vi "RESTful Configure Service Settings.vi"(4 "Number VIs":i32, 6 "Number of Routing Templates":i32, 7 "target reference":refnum<vi>, 8 "error in":errorcluster, 9 "RESTful VI service information":T3, 10 "AMQP Ini In":string="#Service Information", 11 "Master Text In":string="#Service Information") -> (0 "error out":errorcluster, 1 "Service attributes":T1[](array[typedef]), 2 "AMQP Ini Out":string="#Service Information", 3 "Master Text Out":string="#Service Information", 5 "dup target reference":refnum<vi>)   [LabVIEW 2020]
doc: "This VI configure the global settings for the webservices INI file."
uses:
  <vilib>/AppBuilder/Engine/RESTful INI Generator/AB_RESTful_ServiceInfo.ctl
  <vilib>/AppBuilder/AB_Classes/RESTful/AB_RESTful_ServiceAttribute.ctl
  <vilib>/AppBuilder/AB_Classes/RESTful/AB_RESTful_ServiceAttributeType.ctl
  <vilib>/AppBuilder/Engine/RESTful INI Generator/AB_RESTful_ServiceType.ctl
  <vilib>/Utility/error.llb/whitespace.ctl
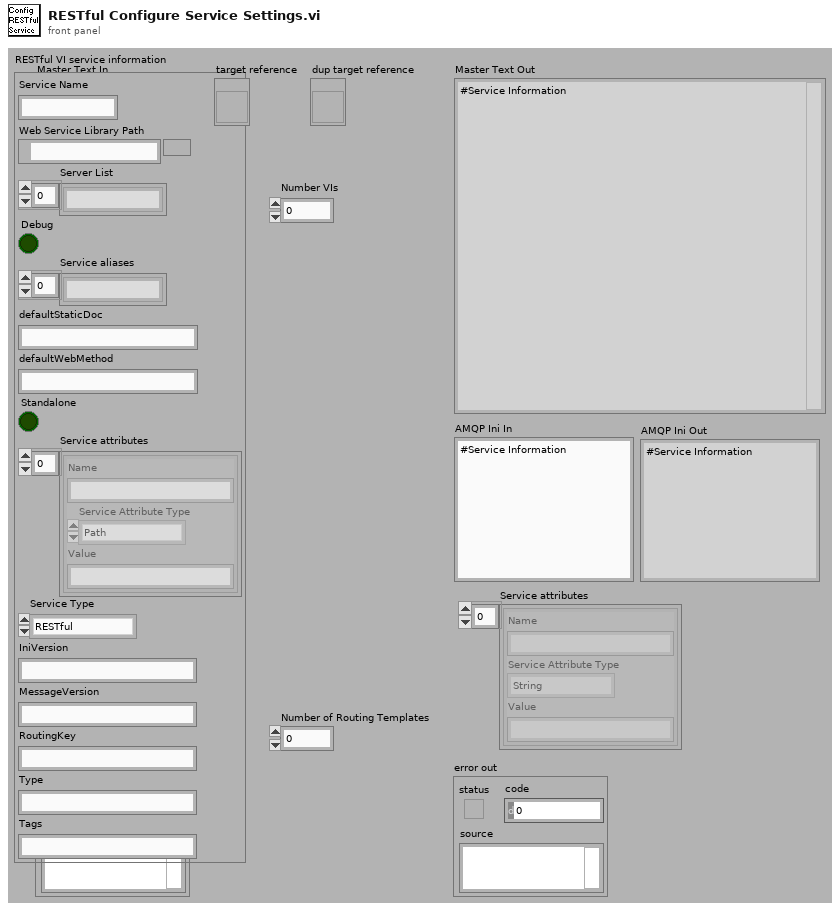
[diagram p1: front panel]
types:
  T1 = typedef "AB_RESTful_ServiceAttribute.ctl" = cluster{"Name":string, "Service Attribute Type":T2, "Value":string}
  T2 = typedef "AB_RESTful_ServiceAttributeType.ctl" = enum32{"String", "Path"}
  T3 = typedef "AB_RESTful_ServiceInfo.ctl" = cluster{"Service Name":string, "Web Service Library Path":path, "Server List":string[], "Debug":bool, "Service aliases":string[], "defaultStaticDoc":string, "defaultWebMethod":string, "Standalone":bool, "Service attributes":T1[], "Service Type":T4, "IniVersion":string, "MessageVersion":string, "RoutingKey":string, "Type":string, "Tags":string}
  T4 = typedef "AB_RESTful_ServiceType.ctl" = enum32{"RESTful", "SOAP", "AMQP"}
  T5 = enum32{"invalid OS target", "Mac OS", "Windows 3.1", "Windows 95/NT", "Solaris 1", "Solaris 2", "HP-UX", "PowerMAX", "Linux", "Irix", "Rhapsody", "BeOS", "AIX", "OSF1", "VxWorks", "PharLap", "Carbon", "RTX", "Windows x64", "Linux x64", "Mac OS X x64"}
  T6 = typedef "whitespace.ctl" = u16
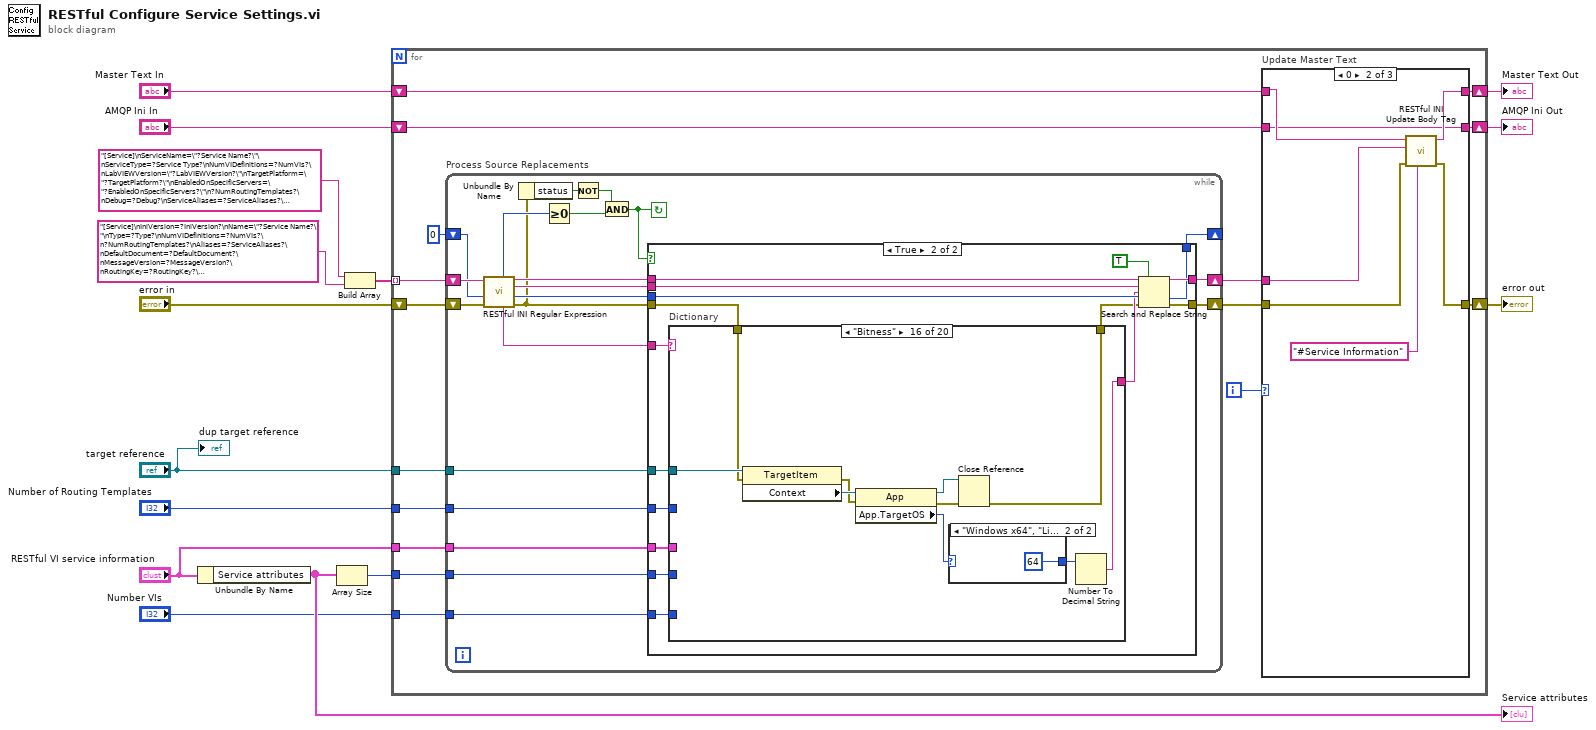
[diagram p0: block diagram]
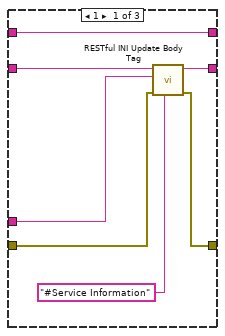
[diagram p2: hidden frame]
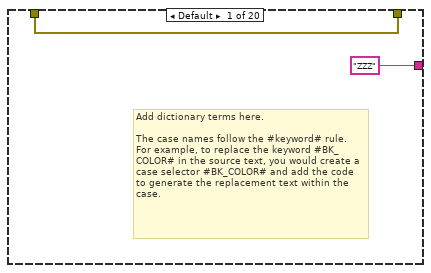
[diagram p5: hidden frame]
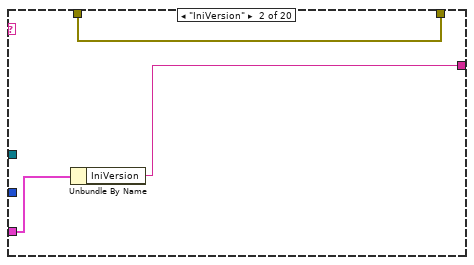
[diagram p6: hidden frame]
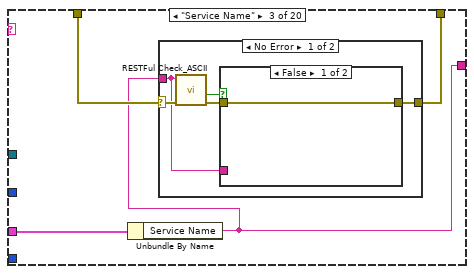
[diagram p7: hidden frame]
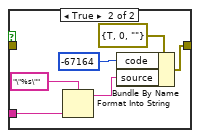
[diagram p8: hidden frame]
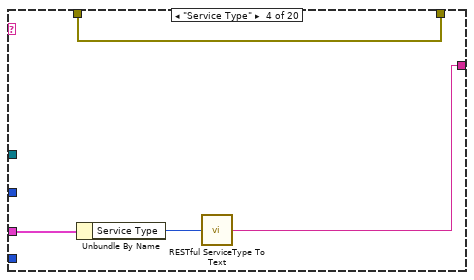
[diagram p10: hidden frame]
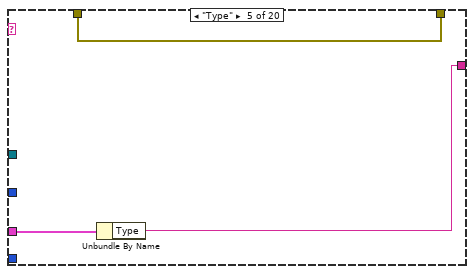
[diagram p11: hidden frame]
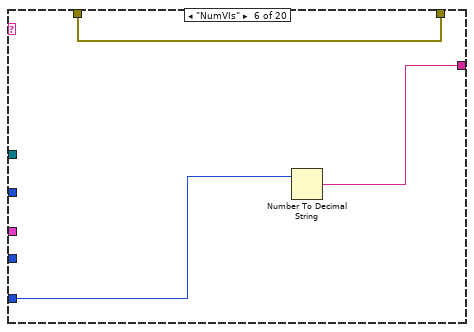
[diagram p12: hidden frame]
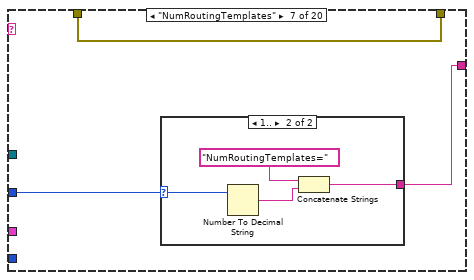
[diagram p13: hidden frame]
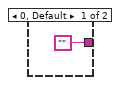
[diagram p14: hidden frame]
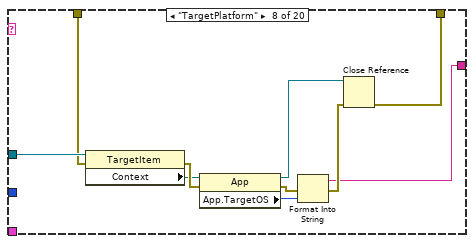
[diagram p15: hidden frame]
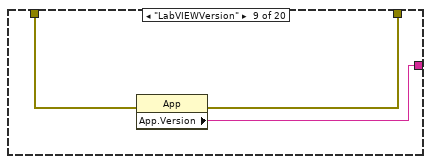
[diagram p16: hidden frame]
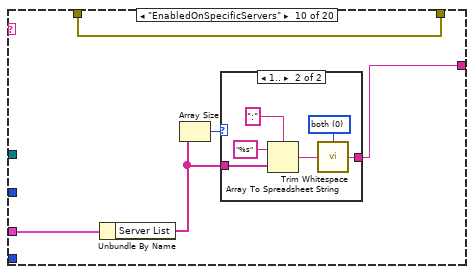
[diagram p17: hidden frame]
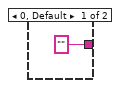
[diagram p18: hidden frame]
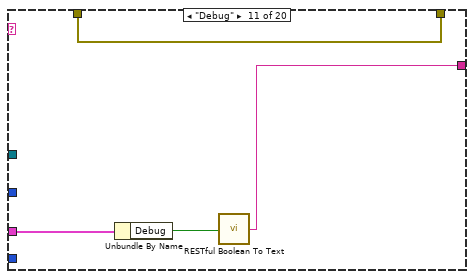
[diagram p19: hidden frame]
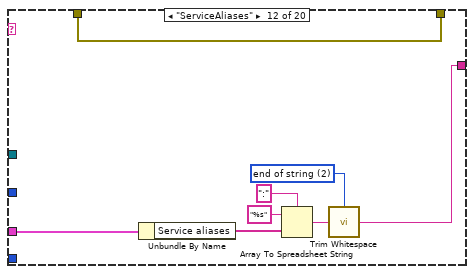
[diagram p20: hidden frame]
diagram:
  n1 = Unbundle By Name("RESTful VI service information") -> ("Service attributes"=w15:T1[])
  "Service attributes" <- w15
  n2 = Array Size(array=w15) -> (size(s)=w9:i32)
  n3 = Build Array("[Service]\nServiceName=\"?Service Name?\"\nServiceType=?Service Type?\nNumVIDefinitions=?NumVIs?\nLabVIEWVersion=\"?LabVIEWVersion?\"\nTargetPlatform=\"?TargetPlatform?\"\nEnabledOnSpecificServers=\"?EnabledOnSpecificServers?\"\n?NumRoutingTemplates?\nDebug=?Debug?\nServiceAliases=?ServiceAliases?\nDefaultDocument=?DefaultDocument?\nDefaultVI=?DefaultVI?\nStandalone=?Standalone?\nBitness=?Bitness?\nNumServiceAttributes=?NumAttributes?", "[Service]\nIniVersion=?IniVersion?\nName=\"?Service Name?\"\nType=?Type?\nNumVIDefinitions=?NumVIs?\n?NumRoutingTemplates?\nAliases=?ServiceAliases?\nDefaultDocument=?DefaultDocument?\nMessageVersion=?MessageVersion?\nRoutingKey=?RoutingKey?\nNumServiceAttributes=?NumAttributes?\nTags=?Tags?") -> (w2:string[])
  n4 = for {
    tunnel: w2 -> [w31] mode=indexing
    shift-right: [w28] -> w4
    shift-left: "AMQP Ini In" -> [w29]
    tunnel: "Number VIs" -> [w27]
    shift-right: [w24] -> w8
    shift-left: "error in" -> [w26]
    tunnel: "Number of Routing Templates" -> [w21]
    tunnel: "RESTful VI service information" -> [w20]
    tunnel: w9 -> [w19]
    shift-right: [w17] -> w5
    shift-left: "Master Text In" -> [w18]
    tunnel: "target reference" -> [w16]
    i -> [w30]
    n5 = while "Process Source Replacements" {
      shift-right: [w64] -> w23
      shift-left: w31 -> [w69]
      tunnel: w27 -> [w63]
      shift-right: [w61] -> w25
      shift-left: w26 -> [w62]
      shift-right: [w60] -> _
      shift-left: 0 ("offset past replacement") -> [w59]
      tunnel: w21 -> [w57]
      tunnel: w20 -> [w56]
      tunnel: w19 -> [w50]
      tunnel: w16 -> [w49]
      stop <- w51 continue-if-true
      n6 = call <vilib>:"RESTful INI Regular Expression.vi"("error in"=w62, "offset (0)"=w59, "input string"=w69) -> ("error out"=w52:errorcluster, "Offset of match"=w66:i32, "whole match"=w65:string, "dup input string"=w67:string, "keyword"=w58:string, "offset past match"=w68:i32)  [unwired: 3 out]
      n7 = Unbundle By Name(w52) -> ("status"=w55:bool)
      n8 = Greater Or Equal To 0?(x=w68) -> (x >= 0?=w53:bool)
      n9 = Not(x=w55) -> (.not. x?=w54:bool)
      n10 = And(x=w54, y=w53) -> (x .and. y?=w51:bool)
      n11 = case shown="True" w51 {
        tunnel: w67 -> [w72 w88]
        tunnel: w66 -> [w70 w87]
        tunnel: w65 -> [_ w86]
        tunnel: [w72 w84] -> w64
        tunnel: w63 -> [_ w83]
        tunnel: [w71 w82] -> w61
        tunnel: w52 -> [w71 w76]
        tunnel: [w70 w81] -> w60
        tunnel: w58 -> [_ w80]
        tunnel: w57 -> [_ w79]
        tunnel: w56 -> [_ w78]
        tunnel: w50 -> [_ w74]
        tunnel: w49 -> [_ w73]
        frame False {
        }
        frame True {
          n12 = case "Dictionary" shown="\"Bitness\"" w80 {
            tunnel: ["ZZZ" w91 w94 w112 w115 w120 w123 w129 w139 w143 w155 w158 w166 w170 w173 w180 w189 w193 w198 w199] -> w85
            tunnel: w83 -> [_ _ _ _ _ w118 _ _ _ _ _ _ _ _ _ _ _ _ _ _]
            tunnel: w79 -> [_ _ _ _ _ _ w122 _ _ _ _ _ _ _ _ _ _ _ _ _]
            tunnel: w78 -> [_ w93 w97 w111 w116 _ _ _ _ w145 w157 w164 w167 w171 w175 _ w190 w195 _ w200]
            tunnel: w76 -> [w89 w92 w96 w114 w117 w119 w121 w131 w141 w144 w154 w165 w168 w169 w172 w184 w188 w194 w197 w201]
            tunnel: [w89 w92 w95 w114 w117 w119 w121 w130 w140 w144 w154 w165 w168 w169 w172 w176 w188 w194 w197 w201] -> w75
            tunnel: w74 -> [_ _ _ _ _ _ _ _ _ _ _ _ _ _ _ _ _ _ w196 _]
            tunnel: w73 -> [_ _ _ _ _ _ _ w132 _ _ _ _ _ _ _ w185 _ _ _ _]
            frame Default {
              # "Add dictionary terms here.\n\nThe case names follow the #keyword# rule.  For example, to replace the keyword #BK_COLOR# in the source text, you would create a case selector #BK_COLOR# and add the code to generate the replacement text within the case."
            }
            frame "IniVersion" {
              n13 = Unbundle By Name(w93) -> ("IniVersion"=w91:string)
            }
            frame "Service Name" {
              n14 = Unbundle By Name(w97) -> ("Service Name"=w94:string)
              n15 = case shown="No Error" w96 {
                selector: w96 -> [w99 w110]
                tunnel: [w100 w110] -> w95
                tunnel: w94 -> [w98 _]
                frame No Error {
                  n16 = call <vilib>:"RESTFul Check_ASCII.vi"("error in (no error)"=w99, "string in"=w98) -> ("error out"=w101:errorcluster, "invalid chars?"=w102:bool)  [unwired: 8 out]
                  n17 = case shown="False" w102 {
                    tunnel: w101 -> [w103 _]
                    tunnel: [w103 w107] -> w100
                    tunnel: w98 -> [_ w104]
                    frame False {
                    }
                    frame True {
                      n18 = Format Into String(format string="\"%s\"", w104) -> (resulting string=w105:string)  [unwired: 2 in, 1 out]
                      n19 = Bundle By Name(cluster=errorcluster {"status"=TRUE, "code"=0, "source"=""} ("error in (no error)"), "code"=-67164 ("error code (0)"), "source"=w105) -> (w107:errorcluster)
                    }
                  }
                }
                frame Error {
                }
              }
            }
            frame "Service Type" {
              n20 = Unbundle By Name(w111) -> ("Service Type"=w113:T4)
              n21 = call <vilib>:"RESTful ServiceType To Text.vi"("Service Type"=w113) -> ("Boolean Text"=w112:string)
            }
            frame "Type" {
              n22 = Unbundle By Name(w116) -> ("Type"=w115:string)
            }
            frame "NumVIs" {
              n23 = Number To Decimal String(number=w118) -> (decimal integer string=w120:string)  [unwired: 1 out]
            }
            frame "NumRoutingTemplates" {
              n24 = case shown="1.." w122 {
                selector: w122 -> [_ w128]
                tunnel: ["" w125] -> w123
                frame 0, Default {
                }
                frame 1.. {
                  n25 = Number To Decimal String(number=w128) -> (decimal integer string=w126:string)  [unwired: 1 out]
                  n26 = Concatenate Strings("NumRoutingTemplates=" ("string"), w126) -> (w125:string)
                }
              }
            }
            frame "TargetPlatform" {
              n27 = property class="TargetItem"(reference=w132, error in=w131) -> (error out=w135:errorcluster, "Context"=w133:refnum<vi>)  [unwired: 1 out]
              n28 = property class="App"(reference=w133, error in=w135) -> (reference out=w138:refnum<vi>, error out=w136:errorcluster, "App.TargetOS"=w134:T5)
              n29 = Format Into String(error in=w136, w134) -> (resulting string=w129:string, error out=w137:errorcluster)  [unwired: 2 in]
              n30 = Close Reference(reference=w138, error in (no error)=w137) -> (error out=w130:errorcluster)
            }
            frame "LabVIEWVersion" {
              n31 = property class="App"(error in=w141) -> (error out=w140:errorcluster, "App.Version"=w139:string)  [unwired: 1 in, 1 out]
            }
            frame "EnabledOnSpecificServers" {
              n32 = Unbundle By Name(w145) -> ("Server List"=w142:string[])
              n33 = Array Size(array=w142) -> (size(s)=w146:i32)
              n34 = case shown="1.." w146 {
                tunnel: ["" ("trimmed string") w150] -> w143
                tunnel: w142 -> [_ w148]
                frame 0, Default {
                }
                frame 1.. {
                  w149 = T6 0 items=["both", "start of string", "end of string"] ("location (both)")
                  n35 = Array To Spreadsheet String(delimiter (Tab)=":", array=w148, 3:"%s" ("format string")) -> (spreadsheet string=w151:string)
                  n36 = call <vilib>:"Trim Whitespace.vi"("string"=w151, "location (both)"=w149) -> ("trimmed string"=w150:string)
                }
              }
            }
            frame "Debug" {
              n37 = Unbundle By Name(w157) -> ("Debug"=w156:bool)
              n38 = call <vilib>:"RESTful Boolean To Text.vi"("Boolean"=w156) -> ("Boolean Text"=w155:string)
            }
            frame "ServiceAliases" {
              w160 = T6 2 items=["both", "start of string", "end of string"] ("location (both)")
              n39 = Unbundle By Name(w164) -> ("Service aliases"=w159:string[])
              n40 = Array To Spreadsheet String(delimiter (Tab)=":", array=w159, 3:"%s" ("format string")) -> (spreadsheet string=w161:string)
              n41 = call <vilib>:"Trim Whitespace.vi"("string"=w161, "location (both)"=w160) -> ("trimmed string"=w158:string)
            }
            frame "DefaultDocument" {
              n42 = Unbundle By Name(w167) -> ("defaultStaticDoc"=w166:string)
            }
            frame "DefaultVI" {
              n43 = Unbundle By Name(w171) -> ("defaultWebMethod"=w170:string)
            }
            frame "Standalone" {
              n44 = Unbundle By Name(w175) -> ("Standalone"=w174:bool)
              n45 = call <vilib>:"RESTful Boolean To Text.vi"("Boolean"=w174) -> ("Boolean Text"=w173:string)
            }
            frame "Bitness" {
              n46 = property class="TargetItem"(reference=w185, error in=w184) -> (error out=w182:errorcluster, "Context"=w183:refnum<vi>)  [unwired: 1 out]
              n47 = property class="App"(reference=w183, error in=w182) -> (reference out=w178:refnum<vi>, error out=w177:errorcluster, "App.TargetOS"=w181:T5)
              n48 = case shown="\"Windows x64\", \"Linux x64\"" w181 {
                tunnel: [32 ("number") 64 ("number")] -> w179
                frame Default {
                }
                frame "Windows x64", "Linux x64" {
                }
              }
              n49 = Close Reference(reference=w178, error in (no error)=w177) -> (error out=w176:errorcluster)
              n50 = Number To Decimal String(number=w179) -> (decimal integer string=w180:string)  [unwired: 1 in]
            }
            frame "MessageVersion" {
              n51 = Unbundle By Name(w190) -> ("MessageVersion"=w189:string)
            }
            frame "RoutingKey" {
              n52 = Unbundle By Name(w195) -> ("Service Name"=w192:string)
              n53 = Concatenate Strings("Skyline.LabVIEWAMQP." ("RutingKey"), w192) -> (w193:string)
            }
            frame "NumAttributes" {
              n54 = Number To Decimal String(number=w196) -> (decimal integer string=w198:string)  [unwired: 1 in]
            }
            frame "Tags" {
              n55 = Unbundle By Name(w200) -> ("Tags"=w199:string)
            }
          }
          n56 = Search and Replace String(replace all?=TRUE ("replace all? (F)"), input string=w88, search string=w86, replace string=w85, offset=w87, error in=w75) -> (result string=w84:string, offset past replacement=w81:i32, error out=w82:errorcluster)  [unwired: 3 out]
        }
      }
    }
    n57 = case "Update Master Text" shown="0" w30 {
      tunnel: w29 -> [w38 w39 w48]
      tunnel: [w37 w39 w48] -> w28
      tunnel: w25 -> [w35 w44 w47]
      tunnel: [w34 w43 w47] -> w24
      tunnel: w23 -> [w36 w45 _]
      tunnel: w18 -> [w32 w41 w46]
      tunnel: [w32 w40 w46] -> w17
      frame 1 {
        n58 = call <vilib>:"RESTful INI Update Body Tag.vi"("Tag"="#Service Information", "error in (no error)"=w35, "Replacement String"=w36, "Input String"=w38) -> ("error out"=w34:errorcluster, "result string"=w37:string)  [unwired: 6 out]
      }
      frame 0 {
        n59 = call <vilib>:"RESTful INI Update Body Tag.vi"("Tag"="#Service Information", "error in (no error)"=w44, "Replacement String"=w45, "Input String"=w41) -> ("error out"=w43:errorcluster, "result string"=w40:string)  [unwired: 6 out]
      }
      frame Default {
      }
    }
  }
  "error out" <- w8
  "Master Text Out" <- w5
  "AMQP Ini Out" <- w4
  "dup target reference" <- "target reference"
